vi "Add Max - Min Data Channels as Fields.vi"(5 "Units":string, 7 "Data Channel":dbl[](array[numeric]), 10 "Channel Name":string, 11 "Fields In":T1[](array[typedef])) -> (3 "Fields Out":T1[](array[typedef]))   [LabVIEW 2011]
uses:
  server/database/Fields/Field Record.ctl
  server/database/Fields/Field DataTypes.ctl
  server/database/Fields/Field NextItem.ctl
  <vilib>/Analysis/NI_AALBase.lvlib
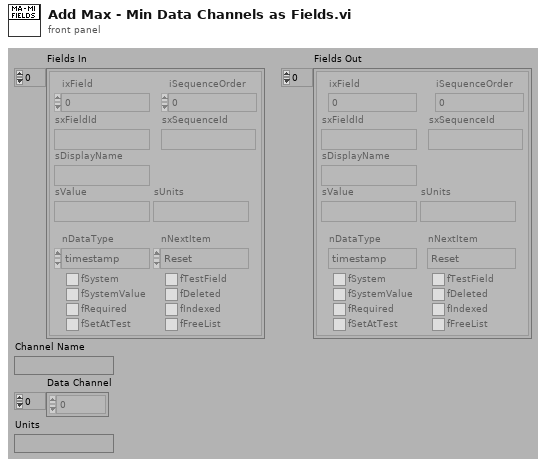
[diagram p1: front panel]
types:
  T1 = typedef "Field Record.ctl" = cluster{"ixField":i32, "iSequenceOrder":i32, "sxFieldId":string, "sxSequenceId":string, "sDisplayName":string, "sValue":string, "sUnits":string, "nDataType":T2, "nNextItem":T3, "fSystem":bool, "fSystemValue":bool, "fRequired":bool, "fSetAtTest":bool, "fTestField":bool, "fDeleted":bool, "fIndexed":bool, "fFreeList":bool}
  T2 = typedef "Field DataTypes.ctl" = enum32{"text", "numeric", "list", "timestamp", "boolean"}
  T3 = typedef "Field NextItem.ctl" = enum32{"Reset", "Retain", "Auto-Increment"}
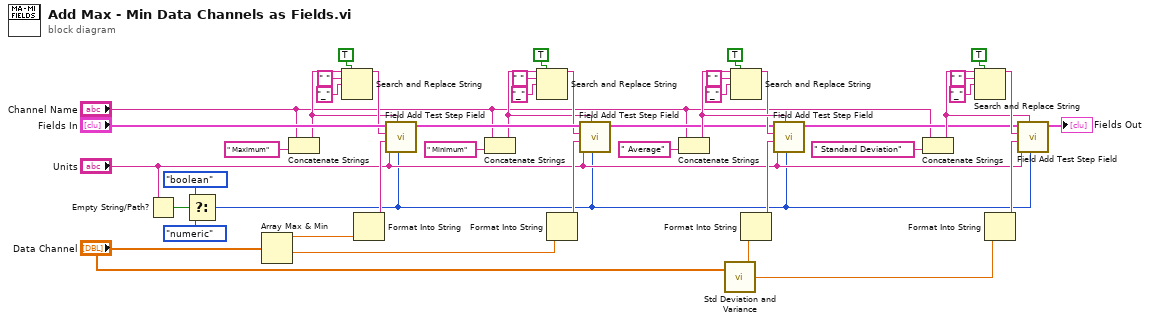
[diagram p0: block diagram]
diagram:
  n1 = Empty String/Path?(string/path="Units") -> (empty?=w36:bool)
  n2 = Select(t=Field_DataTypes."boolean" ("Data Type"), s=w36, f=Field_DataTypes."numeric" ("Data Type")) -> (s? t:f=w5:T2)
  n3 = Array Max & Min(array="Data Channel") -> (max value=w41:dbl, min value=w38:dbl)  [unwired: 2 out]
  n4 = Concatenate Strings("Channel Name", " Maximum" ("string")) -> (w25:string)
  n5 = Search and Replace String(replace all?=TRUE ("replace all? (F)"), input string=w25, search string=" ", replace string="_" ("replace string (\"\")")) -> (result string=w26:string)  [unwired: 1 in, 6 out]
  n6 = Format Into String(w41) -> (resulting string=w42:string)  [unwired: 3 in, 1 out]
  n7 = call "Field Add Test Step Field.vi"("nDataType"=w5, "sDisplayName"=w25, "sUnits"="Units", "sValue"=w42, "sxFieldId"=w26, "Fields In"="Fields In") -> ("Fields Out"=w40:T1[])  [unwired: 5 out]
  n8 = Concatenate Strings("Channel Name", " Minimum" ("string")) -> (w24:string)
  n9 = Search and Replace String(replace all?=TRUE ("replace all? (F)"), input string=w24, search string=" ", replace string="_" ("replace string (\"\")")) -> (result string=w30:string)  [unwired: 1 in, 6 out]
  n10 = Format Into String(w38) -> (resulting string=w39:string)  [unwired: 3 in, 1 out]
  n11 = call "Field Add Test Step Field.vi"("nDataType"=w5, "sDisplayName"=w24, "sUnits"="Units", "sValue"=w39, "sxFieldId"=w30, "Fields In"=w40) -> ("Fields Out"=w7:T1[])  [unwired: 5 out]
  n12 = Concatenate Strings("Channel Name", " Average" ("string")) -> (w23:string)
  n13 = call <vilib>:"Std Deviation and Variance.vi"("X"="Data Channel") -> ("mean"=w2:dbl, "standard deviation"=w3:dbl)  [unwired: 1 in, 1 out]
  n14 = Search and Replace String(replace all?=TRUE ("replace all? (F)"), input string=w23, search string=" ", replace string="_" ("replace string (\"\")")) -> (result string=w22:string)  [unwired: 1 in, 6 out]
  n15 = Format Into String(w2) -> (resulting string=w17:string)  [unwired: 3 in, 1 out]
  n16 = call "Field Add Test Step Field.vi"("nDataType"=w5, "sDisplayName"=w23, "sUnits"="Units", "sValue"=w17, "sxFieldId"=w22, "Fields In"=w7) -> ("Fields Out"=w8:T1[])  [unwired: 5 out]
  n17 = Concatenate Strings("Channel Name", " Standard Deviation" ("string")) -> (w10:string)
  n18 = Search and Replace String(replace all?=TRUE ("replace all? (F)"), input string=w10, search string=" ", replace string="_" ("replace string (\"\")")) -> (result string=w11:string)  [unwired: 1 in, 6 out]
  n19 = Format Into String(w3) -> (resulting string=w16:string)  [unwired: 3 in, 1 out]
  n20 = call "Field Add Test Step Field.vi"("nDataType"=w5, "sDisplayName"=w10, "sUnits"="Units", "sValue"=w16, "sxFieldId"=w11, "Fields In"=w8) -> ("Fields Out"=→"Fields Out":T1[])  [unwired: 5 out]
